vi "calculator.vi"() -> ()   [LabVIEW 2023]
panel:
  in  "stop 2":bool
  in  "DIVISION":bool
  in  "Product":bool
  in  "MINUS":bool
  in  "PLUS":bool
  out "Answer":dbl
  in  "Numeric 2":dbl
  in  "Numeric 1":dbl
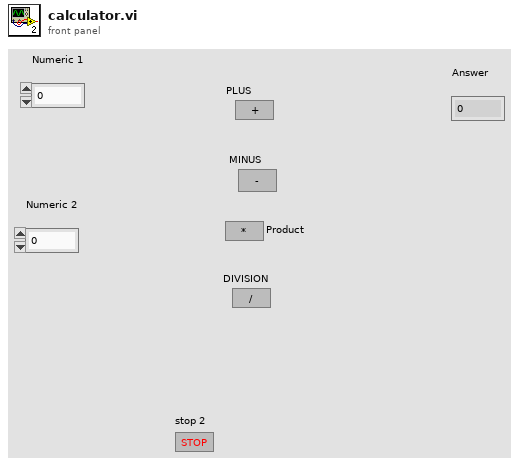
[diagram p1: front panel]
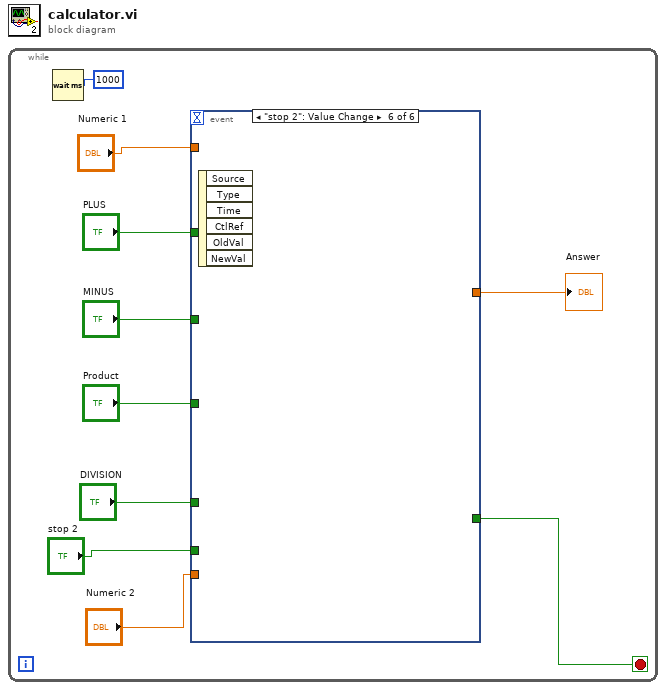
[diagram p0: block diagram]
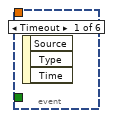
[diagram p2: hidden frame]
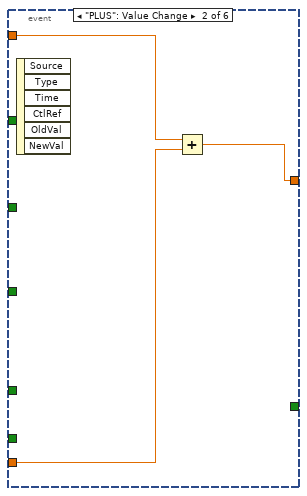
[diagram p3: hidden frame]
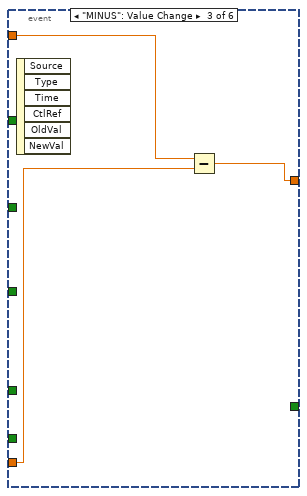
[diagram p4: hidden frame]
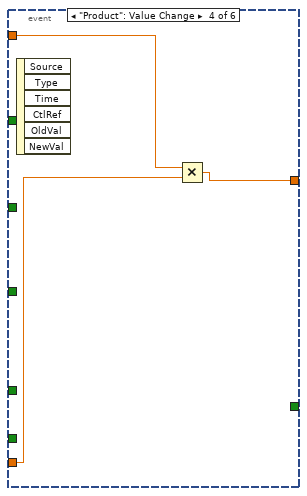
[diagram p5: hidden frame]
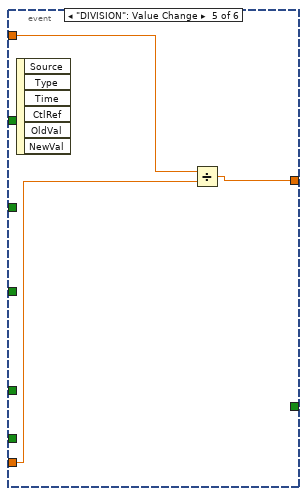
[diagram p6: hidden frame]
diagram:
  n1 = while {
    stop <- w2 stop-if-true
    n2 = Wait (ms)(milliseconds to wait=u32 1000) -> ()  [unwired: 1 out]
    n3 = event shown="[5] \"stop 2\": Value Change" {
      selector: _ -> [_ _ _ _ _ _]
      dyn-events: _ -> [_ _ _ _ _ _]
      timeout: _ -> [_ _ _ _ _ _]
      tunnel: "PLUS" -> [_ _ _ _ _ _]
      tunnel: "MINUS" -> [_ _ _ _ _ _]
      tunnel: "Product" -> [_ _ _ _ _ _]
      tunnel: "DIVISION" -> [_ _ _ _ _ _]
      tunnel: "Numeric 2" -> [_ w12 w15 w18 w21 _]
      tunnel: "Numeric 1" -> [_ w13 w16 w19 w22 _]
      tunnel: [_ w11 w14 w17 w20 _] -> w4
      tunnel: "stop 2" -> [_ _ _ _ _ _]
      tunnel: [_ _ _ _ _ _] -> w2
      event Timeout {
        n4 = event-data() -> ()  [unwired: 1 in, 3 out]
      }
      event "PLUS": Value Change {
        n5 = event-data() -> ()  [unwired: 1 in, 6 out]
        n6 = Add(x=w13, y=w12) -> (x+y=w11:dbl)
      }
      event "MINUS": Value Change {
        n7 = event-data() -> ()  [unwired: 1 in, 6 out]
        n8 = Subtract(x=w16, y=w15) -> (x-y=w14:dbl)
      }
      event "Product": Value Change {
        n9 = event-data() -> ()  [unwired: 1 in, 6 out]
        n10 = Multiply(x=w19, y=w18) -> (x*y=w17:dbl)
      }
      event "DIVISION": Value Change {
        n11 = event-data() -> ()  [unwired: 1 in, 6 out]
        n12 = Divide(x=w22, y=w21) -> (x/y=w20:dbl)
      }
      event "stop 2": Value Change {
        n13 = event-data() -> ()  [unwired: 1 in, 6 out]
      }
    }
    "Answer" <- w4
  }
